vi "Auto_Routine_BlueStraightThreePieceLeftNoteTRAJ.vi"(8 "error in (no error)":errorcluster) -> (0 "error out":errorcluster)   [LabVIEW 2023]
uses:
  Arm2/ArmGetSetpointEnum.ctl
  Trajectory/TrajectoryGlobals.vi
  <vilib>/Rock Robotics/WPI/ThirdParty/JAS_Junk/TrajLib/Trajectory_Library.lvlib
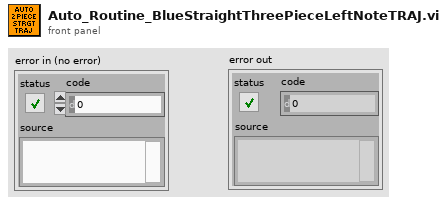
[diagram p1: front panel]
types:
  T1 = typedef "ArmGetSetpointEnum.ctl" = enum16{"ArmFloorPickup", "ArmAmpDeposit", "ArmSpeakerShoot", "ArmStartPosition", "ArmRestPosition", "ArmSourceIntake", "ArmAwayShoot"}
  T2 = typedef "Trajectory_Library.lvlib/TRAJECTORY.ctl" = cluster{"TotalTImeSecs":dbl, "States":T3[]}
  T3 = typedef "Trajectory_Library.lvlib/TRAJ_STATE.ctl" = cluster{"TimeSeconds":dbl, "Velocity":dbl, "Acceleration":dbl, "POSE":T4, "Curvature":dbl}
  T4 = typedef "Trajectory_Library.lvlib/POSE2D.ctl" = cluster{"TRANSLATION":T5, "ROTATION":T6}
  T5 = typedef "Trajectory_Library.lvlib/TRANSLATION2D.ctl" = cluster{"X":dbl, "Y":dbl}
  T6 = typedef "Trajectory_Library.lvlib/ROTATION2D.ctl" = cluster{"VALUE":dbl, "COS":dbl, "SIN":dbl}
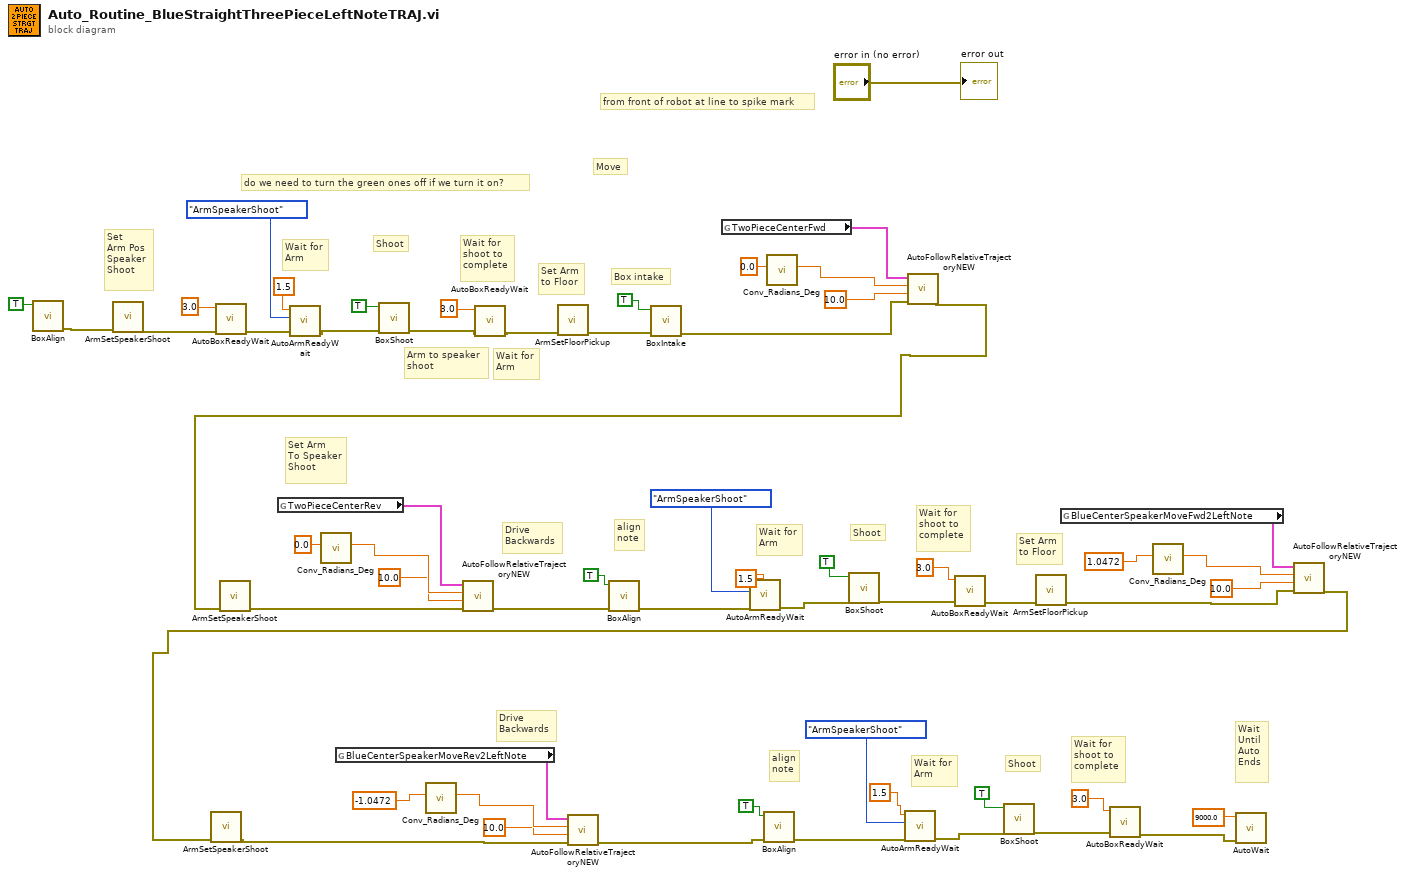
[diagram p0: block diagram]
diagram:
  # "align\nnote"
  # "Wait for\nshoot to\ncomplete"
  # "Shoot"
  # "Wait for\nArm"
  # "Drive\nBackwards"
  # "Set Arm\nto Floor"
  # "align\nnote"
  # "Wait\nUntil\nAuto \nEnds"
  # "Wait for\nshoot to\ncomplete"
  # "Shoot"
  # "Wait for\nArm"
  # "Drive\nBackwards"
  # "Set Arm\nTo Speaker\nShoot"
  # "Wait for\nArm"
  # "Arm to speaker\nshoot"
  # "Box intake"
  # "Move"
  # "Set Arm\nto Floor"
  # "Wait for\nshoot to\ncomplete"
  # "Shoot"
  # "Wait for\nArm"
  # "Set\nArm Pos\nSpeaker\nShoot"
  # "do we need to turn the green ones off if we turn it on?"
  # "from front of robot at line to spike mark"
  n1 = call "BoxAlign.vi"("box align"=TRUE) -> ("error out"=w41:errorcluster)  [unwired: 10 in]
  n2 = call "ArmSetSpeakerShoot.vi"("error in (no error)"=w41) -> ("error out"=w38:errorcluster)  [unwired: 10 in]
  n3 = call "AutoBoxReadyWait.vi"("error in (no error)"=w38, "TimeOut (s)"=3.0) -> ("error out"=w37:errorcluster)  [unwired: 9 in]
  n4 = global read "TrajectoryGlobals.vi" "TwoPieceCenterRev"() -> (w28:T2)
  n5 = call "AutoArmReadyWait.vi"("error in (no error)"=w37, "ArmSetpoints"=ArmGetSetpointEnum."ArmSpeakerShoot", "TimeOut (s)"=1.5) -> ("error out"=w48:errorcluster)  [unwired: 8 in]
  n6 = call <vilib>:"Conv_Radians_Deg.vi"("Radians"=0.0) -> ("Degrees"=w26:dbl)  [unwired: 10 in]
  n7 = global read "TrajectoryGlobals.vi" "BlueCenterSpeakerMoveRev2LeftNote"() -> (w7:T2)
  n8 = call "BoxShoot.vi"("error in (no error)"=w48, "Box shoot"=TRUE) -> ("error out"=w50:errorcluster)  [unwired: 9 in]
  n9 = call <vilib>:"Conv_Radians_Deg.vi"("Radians"=-1.0472) -> ("Degrees"=w5:dbl)  [unwired: 10 in]
  n10 = call "AutoBoxReadyWait.vi"("error in (no error)"=w50, "TimeOut (s)"=3.0) -> ("error out"=w51:errorcluster)  [unwired: 9 in]
  n11 = call "ArmSetFloorPickup.vi"("error in (no error)"=w51) -> ("error out"=w47:errorcluster)  [unwired: 10 in]
  n12 = call "BoxIntake.vi"("error in (no error)"=w47, "Box intake"=TRUE) -> ("error out"=w30:errorcluster)  [unwired: 9 in]
  n13 = global read "TrajectoryGlobals.vi" "TwoPieceCenterFwd"() -> (w34:T2)
  n14 = call <vilib>:"Conv_Radians_Deg.vi"("Radians"=0.0) -> ("Degrees"=w32:dbl)  [unwired: 10 in]
  n15 = call "AutoFollowRelativeTrajectoryNEW.vi"("error in (no error)"=w30, "TimeOut (s)"=10.0, "End Orientation"=w32, "Trajectory"=w34) -> ("error out"=w29:errorcluster)  [unwired: 7 in]
  n16 = call "ArmSetSpeakerShoot.vi"("error in (no error)"=w29) -> ("error out"=w24:errorcluster)  [unwired: 10 in]
  n17 = call "AutoFollowRelativeTrajectoryNEW.vi"("error in (no error)"=w24, "TimeOut (s)"=10.0, "End Orientation"=w26, "Trajectory"=w28) -> ("error out"=w23:errorcluster)  [unwired: 7 in]
  n18 = call "BoxAlign.vi"("error in (no error)"=w23, "box align"=TRUE) -> ("error out"=w35:errorcluster)  [unwired: 9 in]
  n19 = call "AutoArmReadyWait.vi"("error in (no error)"=w35, "ArmSetpoints"=ArmGetSetpointEnum."ArmSpeakerShoot", "TimeOut (s)"=1.5) -> ("error out"=w53:errorcluster)  [unwired: 8 in]
  n20 = call "BoxShoot.vi"("error in (no error)"=w53, "Box shoot"=TRUE) -> ("error out"=w57:errorcluster)  [unwired: 9 in]
  n21 = call "AutoBoxReadyWait.vi"("error in (no error)"=w57, "TimeOut (s)"=3.0) -> ("error out"=w18:errorcluster)  [unwired: 9 in]
  n22 = call "ArmSetFloorPickup.vi"("error in (no error)"=w18) -> ("error out"=w17:errorcluster)  [unwired: 10 in]
  n23 = global read "TrajectoryGlobals.vi" "BlueCenterSpeakerMoveFwd2LeftNote"() -> (w22:T2)
  n24 = call <vilib>:"Conv_Radians_Deg.vi"("Radians"=1.0472) -> ("Degrees"=w20:dbl)  [unwired: 10 in]
  n25 = call "AutoFollowRelativeTrajectoryNEW.vi"("error in (no error)"=w17, "TimeOut (s)"=10.0, "End Orientation"=w20, "Trajectory"=w22) -> ("error out"=w1:errorcluster)  [unwired: 7 in]
  n26 = call "ArmSetSpeakerShoot.vi"("error in (no error)"=w1) -> ("error out"=w3:errorcluster)  [unwired: 10 in]
  n27 = call "AutoFollowRelativeTrajectoryNEW.vi"("error in (no error)"=w3, "TimeOut (s)"=10.0, "End Orientation"=w5, "Trajectory"=w7) -> ("error out"=w2:errorcluster)  [unwired: 7 in]
  n28 = call "BoxAlign.vi"("error in (no error)"=w2, "box align"=TRUE) -> ("error out"=w9:errorcluster)  [unwired: 9 in]
  n29 = call "AutoArmReadyWait.vi"("error in (no error)"=w9, "ArmSetpoints"=ArmGetSetpointEnum."ArmSpeakerShoot", "TimeOut (s)"=1.5) -> ("error out"=w12:errorcluster)  [unwired: 8 in]
  n30 = call "BoxShoot.vi"("error in (no error)"=w12, "Box shoot"=TRUE) -> ("error out"=w15:errorcluster)  [unwired: 9 in]
  n31 = call "AutoBoxReadyWait.vi"("error in (no error)"=w15, "TimeOut (s)"=3.0) -> ("error out"=w8:errorcluster)  [unwired: 9 in]
  n32 = call "AutoWait.vi"("error in (no error)"=w8, "TimeOut (s)"=9000.0) -> ()  [unwired: 9 in, 1 out]
  "error out" <- "error in (no error)"
